vi "Set State.vi"(8 "error in (no error)":errorcluster, 10 "State":T1, 11 "Panel in":refnum<class "Panel.lvclass">) -> (0 "error out":errorcluster, 3 "Panel out":refnum<class "Panel.lvclass">)   [LabVIEW 2020, in "OOPanel.lvlib" / "Panel.lvclass"]
uses:
  Panel.lvclass
  Visibility State.ctl
  OOPanel.lvlib
  Visbility Event Data.ctl
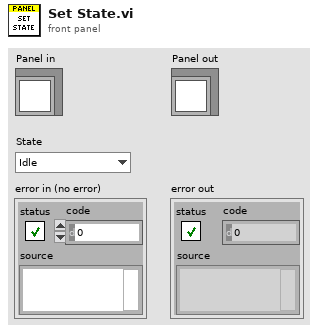
[diagram p1: front panel]
types:
  T1 = typedef "OOPanel.lvlib/Visibility State.ctl" = enum16{"Idle", "Closed", "Hidden", "Visible", "Subpanel", "Hidden Subpanel"}
  T2 = typedef "OOPanel.lvlib/Panel.lvclass/Visbility Event Data.ctl" = cluster{"State":T1}
  T3 = typedef "OOPanel.lvlib/Panel.lvclass/Ref Data.ctl" = cluster{"Panel Ref":refnum<vi>, "SubPanel":refnum<vi>, "Close":bool, "Running":bool, "State":T1}
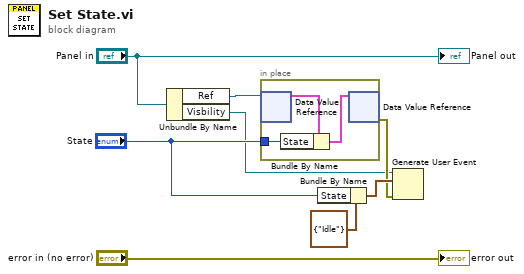
[diagram p0: block diagram]
diagram:
  n1 = Unbundle By Name("Panel in") -> ("Ref"=w7:refnum<data-value>, "Visbility"=w1:refnum<user-event>)
  n2 = in-place {
    in-place-border: "State" -> [w10]
    n3 = in-place-dvr #1(w7) -> (w11:T3)  [unwired: 1 out]
    n4 = Bundle By Name(cluster=w11, "State"=w10) -> (w9:T3)
    n5 = in-place-dvr #1(w9) -> (w2:errorcluster)  [unwired: 1 out]
  }
  n6 = Bundle By Name(cluster=T2 {"State"=enum."Idle"} ("event data"), "State"="State") -> (w4:T2)
  n7 = Generate User Event(user event=w1, event data cluster=w4, error in=w2) -> ()  [unwired: 1 in, 2 out]
  "error out" <- "error in (no error)"
  "Panel out" <- "Panel in"
